vi "State_Machine.vi"(8 "error in (no error)":errorcluster caption="entrée d'erreur (pas d'erreur)", 11 "Get_Voltage en entrée":refnum<class "Zigbee_Read_Msg.lvclass">) -> (0 "error out":errorcluster caption="sortie d'erreur", 2 "Json_String":string, 3 "Get_Voltage en sortie":refnum<class "Zigbee_Read_Msg.lvclass">)   [LabVIEW 2020, in "Library Test.lvlib" / "Zigbee_Read_Msg.lvclass"]
uses:
  Zigbee_Read_Msg.lvclass
  C:/Users/ngarcin/OneDrive - Altyor/Standard TB/Class/Test/Test (Default)/Test (Default).lvclass
  C:/Users/ngarcin/OneDrive - Altyor/Standard TB/Class/Test/Zigbee_Send_Command_UART/Zigbee_Send_Command_UART.lvclass
  JSON API/JSON Value/Set from JSON string.vi
  JSON API/JSON Value/JSON Value.lvclass
  Zigbee_Send_Command_UART/Zigbee_Send_Command_UART.lvclass
  Zigbee_Read_Msg.lvclass/Zigbee_Read_Msg.ctl
  JSON API/Variant JSON/Variant JSON.lvlib
  JSON API/Get Polymorphic/JSON GetSet.lvlib
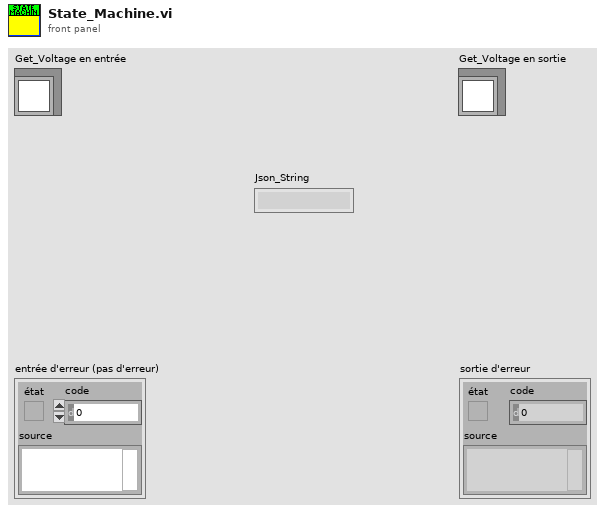
[diagram p1: front panel]
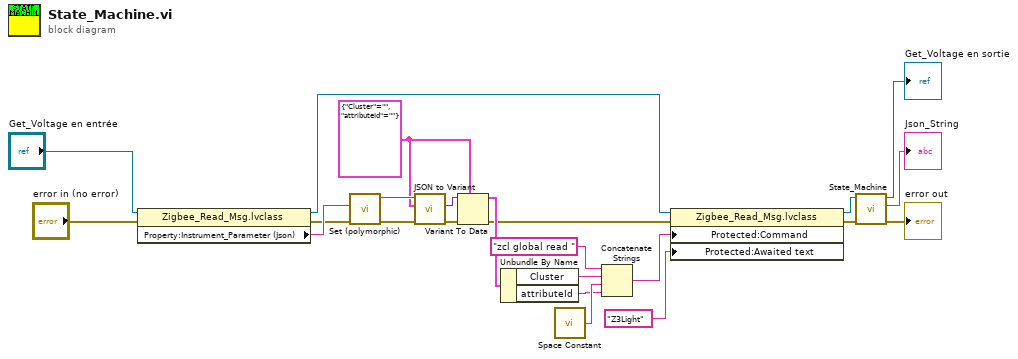
[diagram p0: block diagram]
diagram:
  w12 = cluster{"Cluster":string, "attributeId":string} {"Cluster"="", "attributeId"=""}
  n1 = property class="Zigbee_Read_Msg.lvclass"(reference="Get_Voltage en entrée", error in="error in (no error)") -> (reference out=w7:refnum<class "Zigbee_Read_Msg.lvclass">, error out=w13:errorcluster, "Property:Instrument_Parameter (Json)"=w14:string)
  n2 = call-poly "Set (polymorphic).vi"("error in (no error)"=w13, "JSON stream"=w14) -> ("error out"=w16:errorcluster, "JSON Value out"=w18:refnum<class "JSON Value.lvclass">)  [unwired: 7 in, 1 out]
  n3 = call "JSON to Variant.vi"("error in (no error)"=w16, "Variant (Data Type)"=w12, "JSON Value"=w18) -> ("error out"=w17:errorcluster, "Variant out"=w15:variant)  [unwired: 7 in]
  n4 = Variant To Data(error in=w17, type=w12, Variant=w15) -> (data=w11:cluster{"Cluster":string, "attributeId":string}, error out=w6:errorcluster)
  n5 = Unbundle By Name(w11) -> ("Cluster"=w3:string, "attributeId"=w2:string)
  n6 = call <vilib>:"Space Constant.vi"() -> ("String"=w10:string)
  n7 = Concatenate Strings("zcl global read " ("Command"), w3, w10, w2) -> (w4:string)
  n8 = property class="Zigbee_Read_Msg.lvclass"(reference=w7, error in=w6, "Protected:Command"=w4, "Protected:Awaited text"="Z3Light" ("Awaited text")) -> (reference out=w20:refnum<class "Zigbee_Read_Msg.lvclass">, error out=w19:errorcluster)
  n9 = call-parent "State_Machine.vi"("error in (no error)"=w19, "Send_Frame en entrée"=w20) -> ("error out"=→"error out":errorcluster, "Json_String"=→"Json_String":string, "Send_Frame en sortie"=→"Get_Voltage en sortie":refnum<class "Zigbee_Read_Msg.lvclass">)  [unwired: 7 in]
